vi "Start Event Loop.vi"(10 "Quit Event":refnum<user-event>) -> ()   [LabVIEW 2013, in "Template.lvlib" / "LQCoreEngine.lvclass"]
uses:
  LQCoreEngine.lvclass
  Signal Packet_Void Bool.ctl
  Signal Packet_I32.ctl
  Signal Packet_String.ctl
  Connection Action.ctl
  Template.lvlib
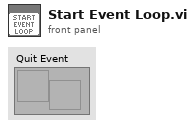
[diagram p1: front panel]
types:
  T1 = typedef "Template.lvlib/LQCoreEngine.lvclass/Signal Packet_String.ctl" = cluster{"QObject Refnum":u64, "Signal Index":i64, "Signal Value":string}
  T2 = typedef "Template.lvlib/LQCoreEngine.lvclass/Signal Packet_I32.ctl" = cluster{"QObject Refnum":u64, "Signal Index":i64, "Signal Value":i32}
  T3 = typedef "Template.lvlib/LQCoreEngine.lvclass/Signal Packet_Void Bool.ctl" = cluster{"QObject Refnum":u64, "Signal Index":i64, "Signal Value":bool}
  T4 = typedef "Template.lvlib/LQCoreEngine.lvclass/Connection Action.ctl" = enum16{"Init", "Add Connection", "Get Connections", "Clean Up"}
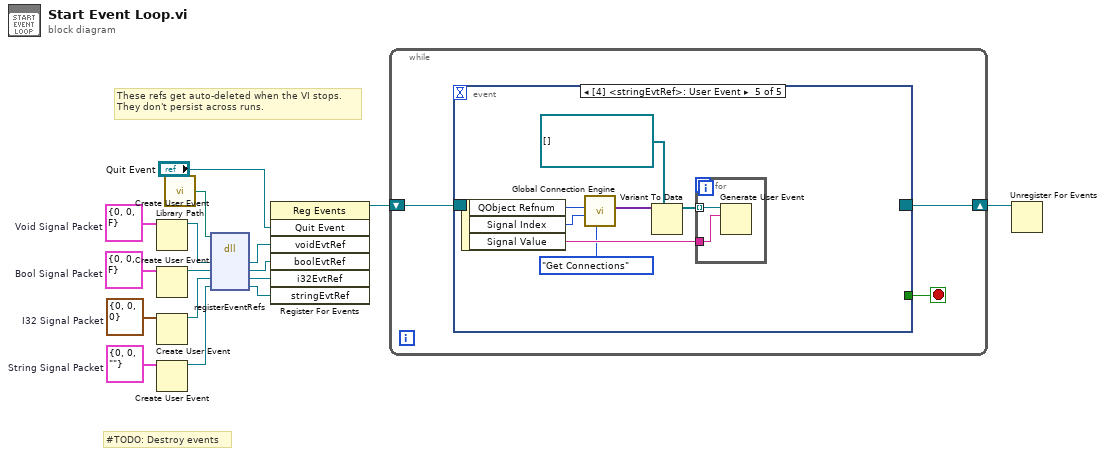
[diagram p0: block diagram]
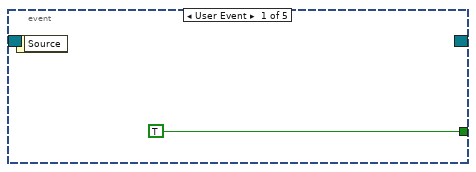
[diagram p2: hidden frame]
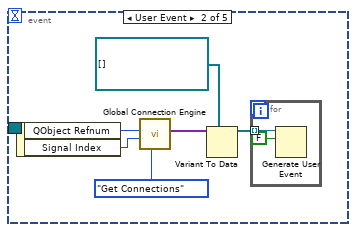
[diagram p3: hidden frame]
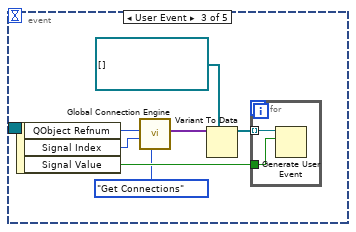
[diagram p4: hidden frame]
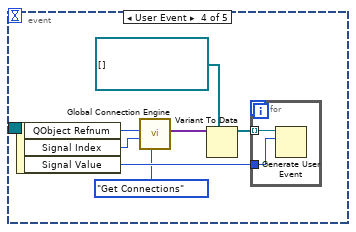
[diagram p5: hidden frame]
diagram:
  w3 = T1 {"QObject Refnum"=0, "Signal Index"=0, "Signal Value"=""}  # String Signal Packet
  w4 = T2 {"QObject Refnum"=0, "Signal Index"=0, "Signal Value"=0}  # I32 Signal Packet
  w5 = T3 {"QObject Refnum"=0, "Signal Index"=0, "Signal Value"=FALSE}  # Bool Signal Packet
  w6 = T3 {"QObject Refnum"=0, "Signal Index"=0, "Signal Value"=FALSE}  # Void Signal Packet
  # "These refs get auto-deleted when the VI stops.\nThey don't persist across runs."
  # "#TODO: Destroy events"
  n1 = Create User Event(user event datatype=w6) -> (user event=w16:refnum<user-event>)  [unwired: 1 in, 1 out]
  n2 = Create User Event(user event datatype=w5) -> (user event=w15:refnum<user-event>)  [unwired: 1 in, 1 out]
  n3 = Create User Event(user event datatype=w4) -> (user event=w14:refnum<user-event>)  [unwired: 1 in, 1 out]
  n4 = Create User Event(user event datatype=w3) -> (user event=w13:refnum<user-event>)  [unwired: 1 in, 1 out]
  n5 = call "Library Path.vi"() -> ("Library Path"=w1:path)
  n6 = dll-call lib="?" fn="registerEventRefs"(path in=w1, "voidEvtRef"=w16, "boolEvtRef"=w15, "i32EvtRef"=w14, "stringEvtRef"=w13) -> ("voidEvtRef"=w12:refnum<user-event>, "boolEvtRef"=w11:refnum<user-event>, "i32EvtRef"=w10:refnum<user-event>, "stringEvtRef"=w9:refnum<user-event>)  [unwired: 3 in, 2 out]
  n7 = register-events("Quit Event", w12, w11, w10, w9) -> (reference out=w8:refnum<event-registration>)  [unwired: 2 in, 1 out]
  n8 = while {
    shift-right: [w18] -> w7
    shift-left: w8 -> [w19]
    stop <- w17 stop-if-true
    n9 = event shown="[4] <stringEvtRef>: User Event" {
      selector: w19 -> [_ _ _ _ _]
      dyn-events: [_ _ _ _ _] -> w18
      timeout: _ -> [_ _ _ _ _]
      tunnel: [TRUE _ _ _ _] -> w17
      event User Event {
        n10 = event-data() -> ()  [unwired: 1 in, 1 out]
      }
      event User Event {
        n11 = event-data() -> ("QObject Refnum"=w23:u64, "Signal Index"=w22:i64)  [unwired: 1 in]
        n12 = call "Global Connection Engine.vi"("Connection Action"=Connection_Action."Get Connections", "Signal Index"=w22, "QObject Refnum"=w23) -> ("Signal Channels"=w26:variant[])  [unwired: 8 in]
        n13 = Variant To Data(type=refnum<user-event>[] [], Variant=w26) -> (data=w24:refnum<user-event>[])  [unwired: 1 in, 1 out]
        n14 = for {
          tunnel: w24 -> [w28] mode=indexing
          n15 = Generate User Event(user event=w28, event data cluster=FALSE ("event data")) -> ()  [unwired: 2 in, 2 out]
        }
      }
      event User Event {
        n16 = event-data() -> ("QObject Refnum"=w35:u64, "Signal Index"=w34:i64, "Signal Value"=w30:bool)  [unwired: 1 in]
        n17 = call "Global Connection Engine.vi"("Connection Action"=Connection_Action."Get Connections", "Signal Index"=w34, "QObject Refnum"=w35) -> ("Signal Channels"=w33:variant[])  [unwired: 8 in]
        n18 = Variant To Data(type=refnum<user-event>[] [], Variant=w33) -> (data=w31:refnum<user-event>[])  [unwired: 1 in, 1 out]
        n19 = for {
          tunnel: w31 -> [w37] mode=indexing
          tunnel: w30 -> [w36]
          n20 = Generate User Event(user event=w37, event data cluster=w36) -> ()  [unwired: 2 in, 2 out]
        }
      }
      event User Event {
        n21 = event-data() -> ("QObject Refnum"=w39:u64, "Signal Index"=w40:i64, "Signal Value"=w41:i32)  [unwired: 1 in]
        n22 = call "Global Connection Engine.vi"("Connection Action"=Connection_Action."Get Connections", "Signal Index"=w40, "QObject Refnum"=w39) -> ("Signal Channels"=w44:variant[])  [unwired: 8 in]
        n23 = Variant To Data(type=refnum<user-event>[] [], Variant=w44) -> (data=w42:refnum<user-event>[])  [unwired: 1 in, 1 out]
        n24 = for {
          tunnel: w42 -> [w46] mode=indexing
          tunnel: w41 -> [w45]
          n25 = Generate User Event(user event=w46, event data cluster=w45) -> ()  [unwired: 2 in, 2 out]
        }
      }
      event User Event {
        n26 = event-data() -> ("QObject Refnum"=w50:u64, "Signal Index"=w49:i64, "Signal Value"=w48:string)  [unwired: 1 in]
        n27 = call "Global Connection Engine.vi"("Connection Action"=Connection_Action."Get Connections", "Signal Index"=w49, "QObject Refnum"=w50) -> ("Signal Channels"=w53:variant[])  [unwired: 8 in]
        n28 = Variant To Data(type=refnum<user-event>[] [], Variant=w53) -> (data=w51:refnum<user-event>[])  [unwired: 1 in, 1 out]
        n29 = for {
          tunnel: w51 -> [w55] mode=indexing
          tunnel: w48 -> [w54]
          n30 = Generate User Event(user event=w55, event data cluster=w54) -> ()  [unwired: 2 in, 2 out]
        }
      }
    }
  }
  n31 = Unregister For Events(event registration refnum=w7) -> ()  [unwired: 1 in, 1 out]
